vi "OP500ZP_PDU.vi"(8 "errin":errorcluster caption="entrée d'erreur (pas d'erreur)") -> (0 "errout":errorcluster caption="sortie d'erreur", 3 "PASS?":bool, 4 "ISO_PDU-":string, 6 "ISO_PDU+":string)   [LabVIEW 2020]
uses:
  OP500ZP_VGConf.vi
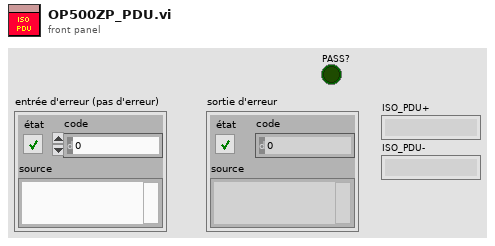
[diagram p1: front panel]
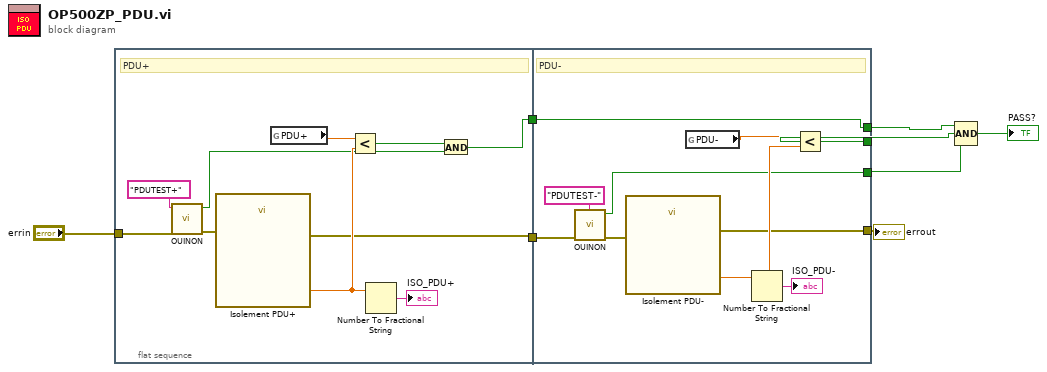
[diagram p0: block diagram]
diagram:
  n1 = flat-sequence {
    tunnel: "errin" -> [w18]
    tunnel: [w12] -> w6
    tunnel: [w9] -> w5
    tunnel: [w26] -> w3
    tunnel: [w22] -> w7
    tunnel: w6 -> [w21]
    tunnel: w5 -> [w20]
    tunnel: [w20] -> w4
    tunnel: [w19] -> w2
    frame #0 {
      # "PDU+"
      n2 = call <userlib>:"OUINON.vi"("errin"=w18, "image"="PDUTEST+") -> ("error out"=w17:errorcluster, "OUI/NON"=w11:bool)  [unwired: 8 in]
      n3 = call "Isolement PDU+"("error in (no error)"=w17) -> ("ISO_PDU+"=w15:dbl, "error out"=w12:errorcluster)  [unwired: 16 in, 1 out]
      n4 = global read "OP500ZP_VGConf.vi" "PDU+"() -> (w13:dbl)
      n5 = Less?(x=w13, y=w15) -> (x < y?=w10:bool)
      n6 = Number To Fractional String(number=w15) -> (F-format string=→"ISO_PDU+":string)  [unwired: 3 in]
      n7 = And(x=w10, y=w11) -> (x .and. y?=w9:bool)
    }
    frame #1 {
      # "PDU-"
      n8 = call <userlib>:"OUINON.vi"("errin"=w21, "image"="PDUTEST-") -> ("error out"=w27:errorcluster, "OUI/NON"=w19:bool)  [unwired: 8 in]
      n9 = call "Isolement PDU-"("error in (no error)"=w27) -> ("ISO_PDU-"=w25:dbl, "error out"=w22:errorcluster)  [unwired: 16 in, 1 out]
      n10 = global read "OP500ZP_VGConf.vi" "PDU-"() -> (w23:dbl)
      n11 = Number To Fractional String(number=w25) -> (F-format string=→"ISO_PDU-":string)  [unwired: 3 in]
      n12 = Less?(x=w23, y=w25) -> (x < y?=w26:bool)
    }
  }
  n13 = Compound Arithmetic op=AND ("Opérateur arithmétique")(w4, w3, w2) -> (→"PASS?":bool)
  "errout" <- w7
